vi "DB. Select.vi"(0 "conn ref":T1, 5 "SQL query":string="SELECT distinct EN_ID, MODEL FROM asti_wh_management.cm_source_data where EN_ID = 4634", 11 "error in (no error)":errorcluster) -> (4 "conn ref 2":T1, 6 "recordset data":variant[][](array[variant]), 8 "data":string[][](array[string]), 10 "NULL":bool, 15 "error out":errorcluster)   [LabVIEW 2015]
uses:
  <vilib>/addons/database/Connection.llb/Conn ObjectReference.ctl
  <vilib>/addons/database/Connection.llb/Conn Execute.vi
  <vilib>/addons/database/Recordset.llb/Rec Fetch Recordset Data (R).vi
  <vilib>/addons/database/Recordset.llb/Rec Destroy - Connection.vi
  <vilib>/addons/database/_DB Variant To Data/Database Variant To Data.xnode
  <vilib>/addons/database/NI_Database_API.lvlib
  <vilib>/addons/database/Connection.llb/Conn Properties.ctl
  <vilib>/addons/database/Connection.llb/Conn Set Properties.vi
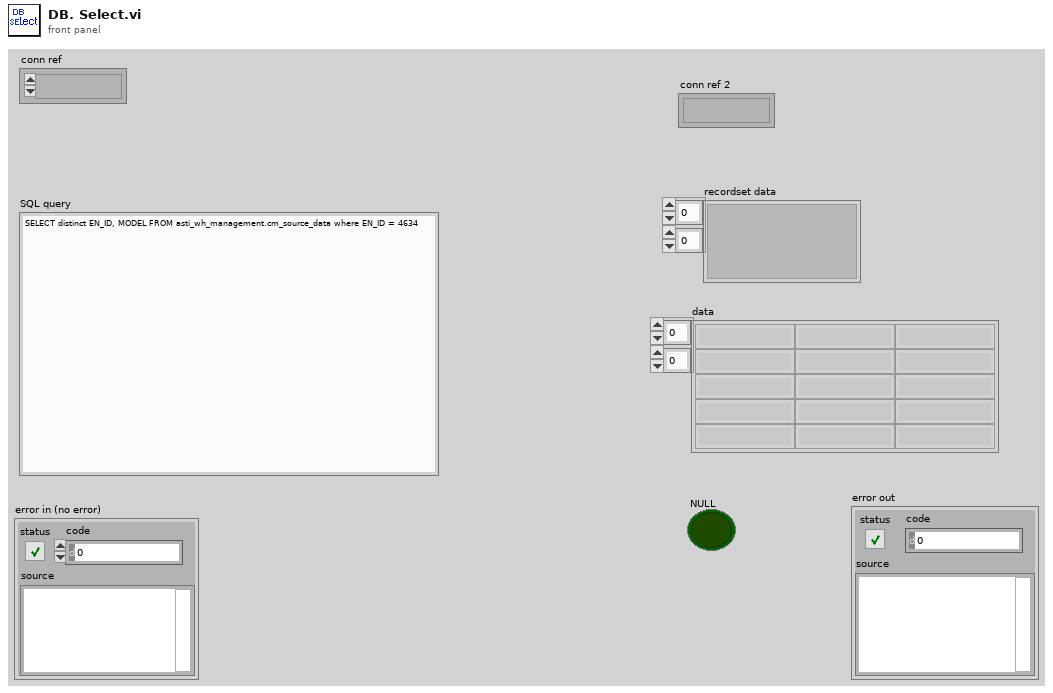
[diagram p1: front panel]
types:
  T1 = typedef "NI_Database_API.lvlib/Conn ObjectReference.ctl" = refnum<k1>
  T2 = typedef "NI_Database_API.lvlib/Conn Properties.ctl" = cluster{"command timeout (s)":i32, "connection string":string, "default database":string, "provider":string}
  T3 = typedef "NI_Database_API.lvlib/Rec ObjectReference.ctl" = refnum<k1>
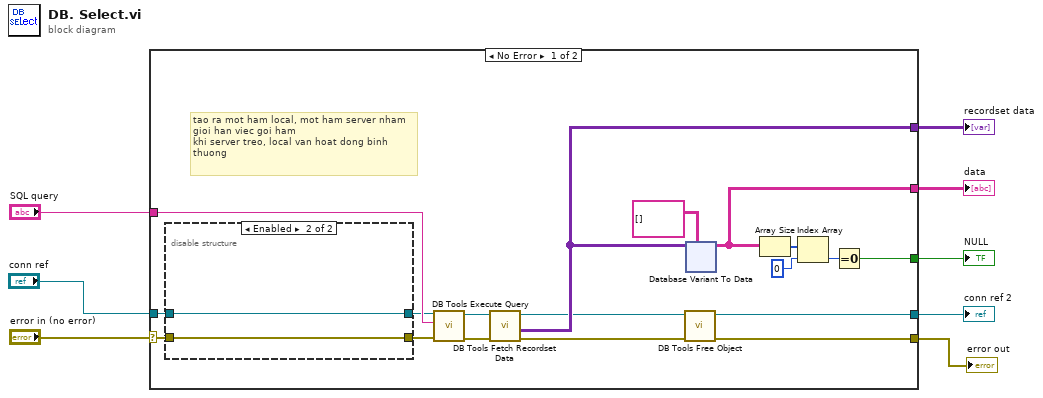
[diagram p0: block diagram]
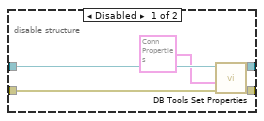
[diagram p2: hidden frame]
diagram:
  n1 = case shown="No Error" "error in (no error)" {
    selector: "error in (no error)" -> [w12 w79]
    tunnel: [w26 w79] -> w2
    tunnel: "SQL query" -> [w23 _]
    tunnel: [w22 _] -> w7
    tunnel: [w20 _] -> w6
    tunnel: [w16 _] -> w5
    tunnel: [w15 w78] -> w3
    tunnel: "conn ref" -> [w13 w78]
    frame No Error {
      # "tao ra mot ham local, mot ham server nham gioi han viec goi ham\nkhi server treo, local van hoat dong binh thuong"
      n2 = disable-structure shown="Enabled" {
        disable-tunnel: [w31 w33] -> w14
        disable-tunnel: w13 -> [w30 w33]
        disable-tunnel: w12 -> [w29 w32]
        disable-tunnel: [w28 w32] -> w11
        frame Disabled {
          n3 = call-poly <vilib>:"DB Tools Set Properties.vi"("error in (no error)"=w29, "connection properties"=T2 {"command timeout (s)"=15, "connection string"="", "default database"="asti_wh_management", "provider"=""}, "connection reference"=w30) -> ("error out"=w28:errorcluster, "connection reference out"=w31:T1)  [unwired: 3 in]
        }
        frame Enabled {
        }
      }
      n4 = call-poly <vilib>:"DB Tools Execute Query.vi"("error in (no error)"=w11, "SQL query"=w23, "connection reference"=w14) -> ("error out"=w24:errorcluster, "recordset reference"=w25:T3)  [unwired: 5 in]
      n5 = call-poly <vilib>:"DB Tools Fetch Recordset Data.vi"("error in (no error)"=w24, "recordset reference"=w25) -> ("error out"=w9:errorcluster, "recordset data"=w22:variant[][], "recordset reference out"=w10:T3)  [unwired: 3 in]
      n6 = call-poly <vilib>:"DB Tools Free Object.vi"("error in (no error)"=w9, "recordset reference"=w10) -> ("error out"=w26:errorcluster, "connection reference"=w15:T1)  [unwired: 8 in]
      n7 = xnode "Database Variant To Data"("database variant"=w22, "type"=string[][] [] ("array")) -> ("data"=w20:string[][])  [unwired: 1 in, 1 out]
      n8 = Array Size(array=w20) -> (size(s)=w19:i32[])
      n9 = Index Array(array=w19, index=0) -> (element=w17:i32)
      n10 = Equal To 0?(x=w17) -> (x = 0?=w16:bool)
    }
    frame Error {
    }
  }
  "error out" <- w2
  "data" <- w6
  "NULL" <- w5
  "recordset data" <- w7
  "conn ref 2" <- w3
